vi "Iteration Memory.vi"() -> ()   [LabVIEW 2020]
panel:
  in  "stop":bool
  out "Current":dbl
  out "Three Iter Ago":dbl
  out "Two Iter Ago":dbl
  out "Previous Count":dbl
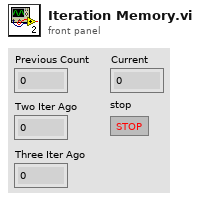
[diagram p1: front panel]
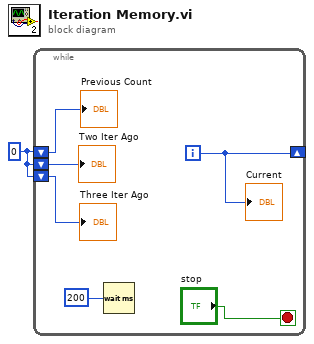
[diagram p0: block diagram]
diagram:
  w1 = 0
  n1 = while {
    shift-right: [w6] -> _
    shift-left: w1 -> [w4]
    shift-left: w1 -> [w2]
    shift-left: w1 -> [w3]
    i -> [w6]
    stop <- "stop" stop-if-true
    n2 = Wait (ms)(milliseconds to wait=u32 200 ("millisecond timer value")) -> ()  [unwired: 1 out]
    "Previous Count" <- w4
    "Two Iter Ago" <- w3
    "Three Iter Ago" <- w2
    "Current" <- w6
  }
